vi "Initialize DeepU Panel.vi"() -> (0 "error out":errorcluster, 2 "DeepU Results queue out":refnum<queue>, 3 "Event Registration Refnum":refnum<event-registration>)   [LabVIEW 2019, in "Test Stands.lvlib" / "DeepU Test Stand.lvclass"]
uses:
  DeepU Test Stand.lvclass
  C:/Users/wg/Documents/LV_Projects/test-stand/App/Generic Test Stand/Generic Test Stand.lvclass
  Generic Test Stand/Generic Test Stand.lvclass/Generic Test Stand.ctl
  DeepU Test Stand.lvclass/DeepU Test Stand.ctl
  Generic Test Stand/Generic Test Stand.lvclass
  Results/DeepU Results/DeepU Results.lvclass
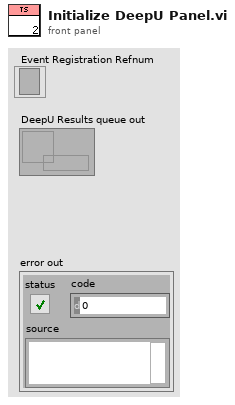
[diagram p1: front panel]
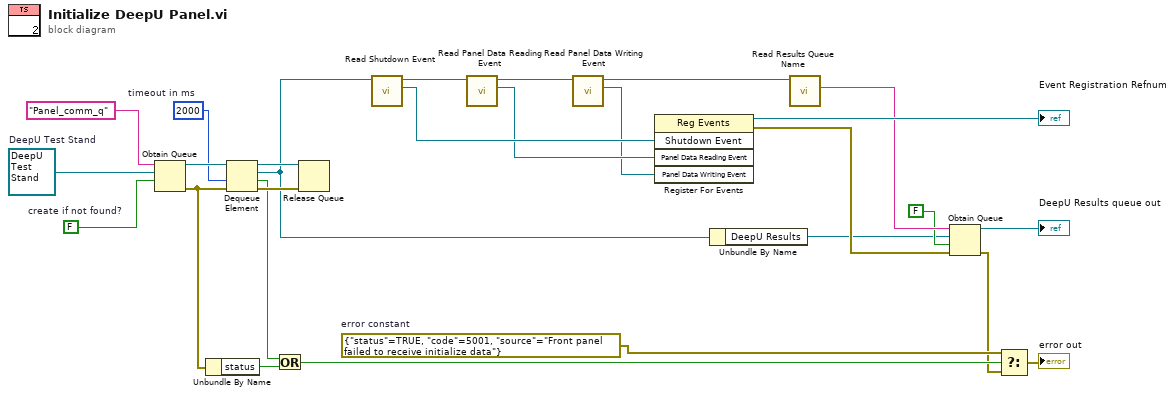
[diagram p0: block diagram]
diagram:
  w5 = refnum<class "DeepU Test Stand.lvclass"> refnum  # DeepU Test Stand
  w11 = errorcluster {"status"=TRUE, "code"=5001, "source"="Front panel failed to receive initialize data"}  # error constant
  w24 = 2000  # timeout in ms
  w26 = FALSE  # create if not found?
  n1 = Obtain Queue(name (unnamed)="Panel_comm_q", element data type=w5, create if not found? (T)=w26) -> (queue out=w25:refnum<queue>, error out=w15:errorcluster)  [unwired: 2 in, 1 out]
  n2 = Unbundle By Name(w15) -> ("status"=w14:bool)
  n3 = Dequeue Element(queue=w25, timeout in ms (-1)=w24, error in (no error)=w15) -> (queue out=w23:refnum<queue>, element=w3:refnum<class "DeepU Test Stand.lvclass">, timed out?=w13:bool, error out=w22:errorcluster)
  n4 = Or(x=w13, y=w14) -> (x .or. y?=w12:bool)
  n5 = Release Queue(queue=w23, error in (no error)=w22) -> ()  [unwired: 1 in, 3 out]
  n6 = call "Read Shutdown Event.vi"("Generic Test Stand in"=w3) -> ("Shutdown Event"=w21:refnum<user-event>, "Generic Test Stand out"=w20:refnum<class "DeepU Test Stand.lvclass">)  [unwired: 8 in, 1 out]
  n7 = call "Read Panel Data Reading Event.vi"("Generic Test Stand in"=w20) -> ("Panel Data Reading Event"=w18:refnum<user-event>, "Generic Test Stand out"=w19:refnum<class "DeepU Test Stand.lvclass">)  [unwired: 8 in, 1 out]
  n8 = call "Read Panel Data Writing Event.vi"("Generic Test Stand in"=w19) -> ("Panel Data Writing Event"=w17:refnum<user-event>, "Generic Test Stand out"=w4:refnum<class "DeepU Test Stand.lvclass">)  [unwired: 8 in, 1 out]
  n9 = register-events(w21, w18, w17) -> (reference out=→"Event Registration Refnum":refnum<event-registration>, error out=w6:errorcluster)  [unwired: 2 in]
  n10 = Unbundle By Name(w3) -> ("DeepU Results"=w2:refnum<class "DeepU Results.lvclass">)
  n11 = call "Read Results Queue Name.vi"("Generic Test Stand in"=w4) -> ("Results Queue Name"=w9:string)  [unwired: 8 in, 2 out]
  n12 = Obtain Queue(name (unnamed)=w9, element data type=w2, create if not found? (T)=FALSE, error in (no error)=w6) -> (queue out=→"DeepU Results queue out":refnum<queue>, error out=w7:errorcluster)  [unwired: 1 in, 1 out]
  n13 = Select(t=w11, s=w12, f=w7) -> (s? t:f=→"error out":errorcluster)
